vi "Read XML Document.lvclass.vi"(8 "error in":errorcluster, 11 "XML Editor GUI in":refnum<class "XML Editor GUI.lvclass">) -> (0 "error out":errorcluster, 2 "XML Document.lvclass":refnum<class "XML Document.lvclass">, 3 "XML Editor GUI out":refnum<class "XML Editor GUI.lvclass">)   [LabVIEW 2014, in "XML Editor GUI.lvclass"]
uses:
  XML Editor GUI.lvclass
  XML Document_class/XML Document.lvclass
  XML Editor GUI.lvclass/XML Editor GUI.ctl
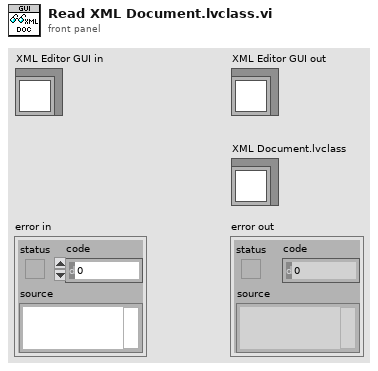
[diagram p1: front panel]
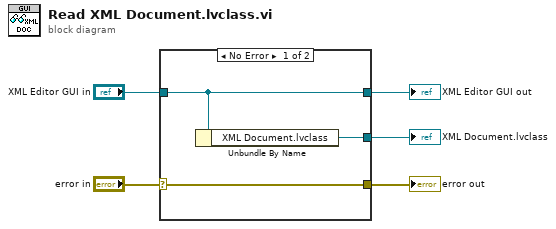
[diagram p0: block diagram]
diagram:
  n1 = case shown="No Error" "error in" {
    selector: "error in" -> [w8 w9]
    tunnel: [w8 w9] -> w4
    tunnel: [w7 w10] -> w2
    tunnel: "XML Editor GUI in" -> [w7 w10]
    tunnel: [w6 _] -> w1
    frame No Error {
      n2 = Unbundle By Name(w7) -> ("XML Document.lvclass"=w6:refnum<class "XML Document.lvclass">)
    }
    frame Error {
    }
  }
  "error out" <- w4
  "XML Editor GUI out" <- w2
  "XML Document.lvclass" <- w1
